vi "PosStrikerAnguloGolV1.vi"(8 "AnguloAttacker":dbl, 9 "atacando contra":bool, 10 "IA State":T1={"our_robots"=[], "enemy_robots"=[], "balls"=[], "geometry"={"line_width"=0, "field_length"=0, "field_width"=0, "boundary_width"=0, "referee_width"=0, "goal_width"=0, "goal_depth"=0, "goal_wall_width"=0, "center_circle_radius"=0, "defense_radius"=0, "defense_stretch"=0, "free_kick_from_defense_dist"=0, "penalty_spot_from_field_line_dist"=0, "penalty_line_from_spot_dist"=0}, "IA Judge"={"stage"="", "command"="", "our_goalie_id"=0.0, "enemy_goalie_id"=0.0, "command enum"=enum."Halt", "Time"=enum."Azul"}, "Received Timestamp"=timestamp(0 s since 1904-01-01), "Events"={"Touch"=FALSE, "Ball out"=FALSE, "id touch"=0.0, "Ball out of \nVision"=FALSE, "Ball inside \nGoalie area"=FALSE, "Robot not responding"=FALSE, "Robots responding status"=[1.0, 1.0, 1.0, 1.0, 1.0, 1.0], "Enemy Ball \nPossession"=FALSE, "Pass State"=FALSE, "id end of pass"=0.0, "Kick"=FALSE, "Id ini Possession"=0.0, "Ball Possesion"=FALSE, "Id Possesion"=0.0, "Direct Kick"=FALSE, "2nd Strk Ativo"=FALSE}}) -> (2 "theta final":dbl)   [LabVIEW 2017]
uses:
  Core/AI Input.ctl
  Core/AI Robot.ctl
  Intel/Functions Enum.ctl
  Intel/AttackerStates.ctl
  Path Planning/RRT/PathDests.ctl
  Path Planning/RRT/PathDest.ctl
  Core/AI Ball.ctl
  Core/Field Size.ctl
  Core/AI Judge.ctl
  Intel/Command Enum.ctl
  Events/Events.ctl
panel:
  in  "XdoAttacker":dbl
  in  "YdoAttacker":dbl
  in  "Array":dbl[](array[numeric])=[0.0, 0.0, 0.0, 0.0, 0.0, 0.0]
  in  "Contador 2":dbl
  in  "theta2":dbl=-1.57
  in  "inicio do intervalo":dbl=-1.57
  in  "tamanho do intervalo":dbl
  in  "valor de theta":dbl
  in  "RobôsParaAnalisar":dbl[][](array[numeric])=[[99999.0, 99999.0], [99999.0, 99999.0], [99999.0, 99999.0], [99999.0, 99999.0], [99999.0, 99999.0], [99999.0, 99999.0], [99999.0, 99999.0]]
  in  "Contador":dbl
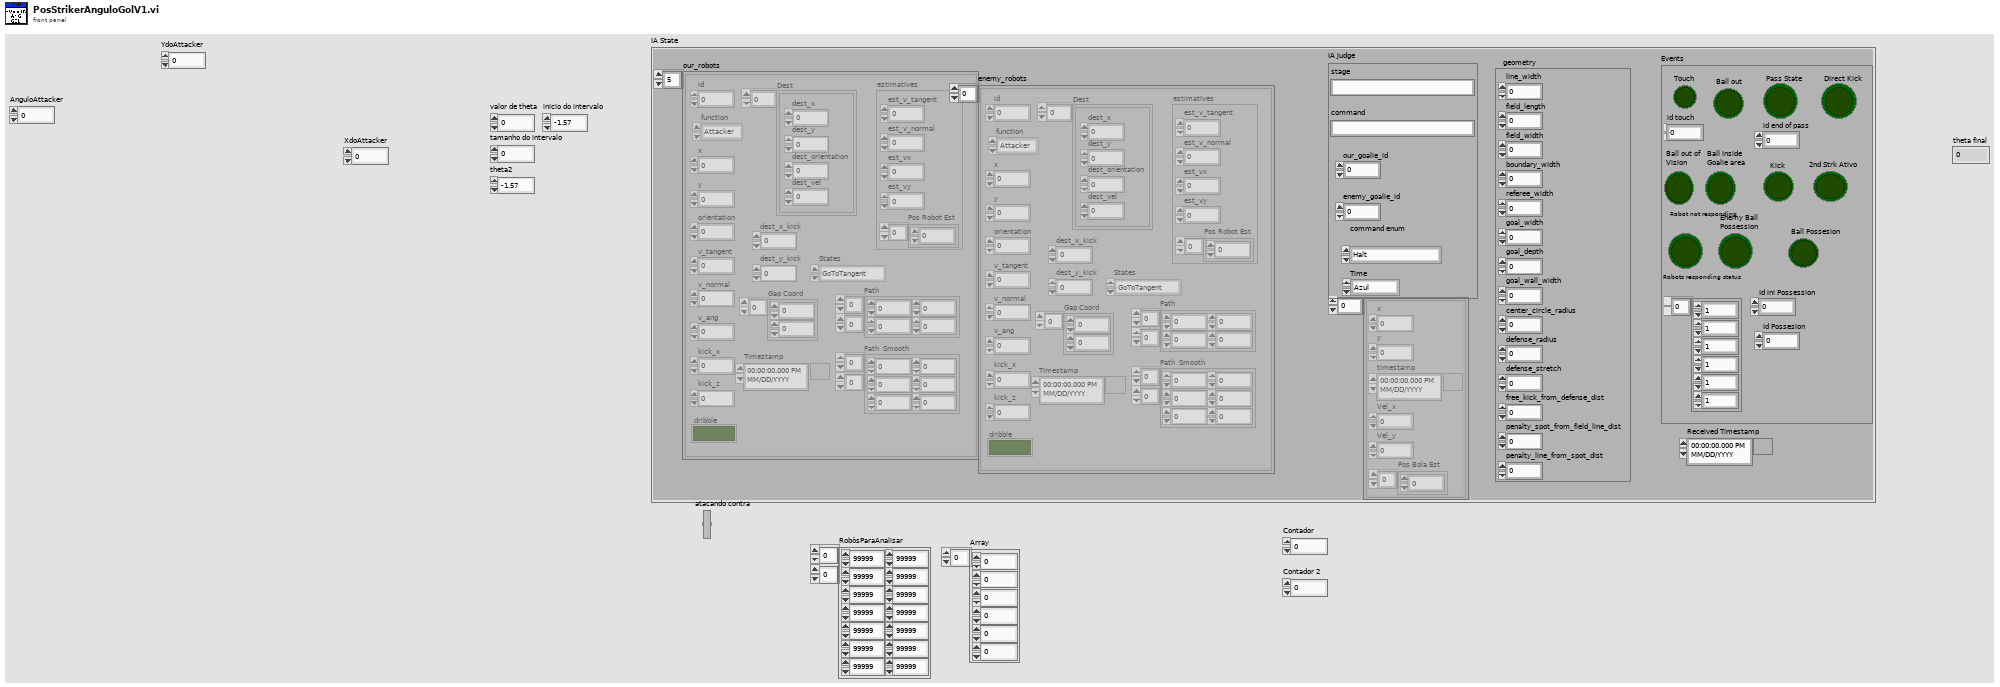
[diagram p1: front panel]
types:
  T1 = typedef "AI Input.ctl" = cluster{"our_robots":T2[], "enemy_robots":T2[], "balls":T7[], "geometry":T8, "IA Judge":T9, "Received Timestamp":timestamp, "Events":T11}
  T2 = typedef "AI Robot.ctl" = cluster{"id":u32, "function":T3, "x":dbl, "y":dbl, "orientation":dbl, "v_tangent":dbl, "v_normal":dbl, "v_ang":dbl, "kick_x":dbl, "kick_z":dbl, "dribble":bool, "Timestamp":timestamp, "estimatives":cluster{"est_v_tangent":dbl, "est_v_normal":dbl, "est_vx":dbl, "est_vy":dbl, "Pos Robot Est":dbl[]}, "dest_x_kick":dbl, "dest_y_kick":dbl, "Gap Coord":dbl[], "States":T4, "Path ":dbl[][], "Path  Smooth":dbl[][], "Dest":T5}
  T3 = typedef "Functions Enum.ctl" = enum16{"2nd Striker", "Attacker", "Goalie", "Defender", "Striker", "Goto 0", "Dummy", "Kicker", "ZigZag 0", "ZigZag 1", "ZigZag 2", "ZigZag 3", "ZigZag 4", "ZigZag 5", "ZigZag 6", "ZigZag 7", "ZigZag 8", ""}
  T4 = typedef "AttackerStates.ctl" = enum16{"Pass", "GoToTangent", "BallGetting", "GoToKick", ""}
  T5 = typedef "PathDests.ctl" = T6[]
  T6 = typedef "PathDest.ctl" = cluster{"dest_x":dbl, "dest_y":dbl, "dest_orientation":dbl, "dest_vel":dbl}
  T7 = typedef "AI Ball.ctl" = cluster{"x":dbl, "y":dbl, "timestamp":timestamp, "Vel_x":dbl, "Vel_y":dbl, "Pos Bola Est":dbl[]}
  T8 = typedef "Field Size.ctl" = cluster{"line_width":u32, "field_length":u32, "field_width":u32, "boundary_width":u32, "referee_width":u32, "goal_width":u32, "goal_depth":u32, "goal_wall_width":u32, "center_circle_radius":u32, "defense_radius":u32, "defense_stretch":u32, "free_kick_from_defense_dist":u32, "penalty_spot_from_field_line_dist":u32, "penalty_line_from_spot_dist":u32}
  T9 = typedef "AI Judge.ctl" = cluster{"stage":string, "command":string, "our_goalie_id":dbl, "enemy_goalie_id":dbl, "command enum":T10, "Time":enum16{"Azul", "Amarelo"}}
  T10 = typedef "Command Enum.ctl" = enum16{"Halt", "Stop", "Force Start", "PKA Normal Start", "Prepare Kickoff Ally", "PKE Normal Start", "Prepare Kickoff Enemy", "Prepare Penalty Ally", "PPA Normal Start", "Prepare Penalty Enemy", "PPE Normal Start", "Direct Free Enemy", "Direct Free Ally", "Indirect Free Enemy", "Indirect Free Ally", "Timeout Enemy", "Timeout Ally", "Goal Enemy", "Goal Ally", "Ball Placement Enemy", "Ball Placement Ally", "Normal Half Time", "Extra Time Break", "Extra Half Time", "None", "Post Game"}
  T11 = typedef "Events.ctl" = cluster{"Touch":bool, "Ball out":bool, "id touch":dbl, "Ball out of \nVision":bool, "Ball inside \nGoalie area":bool, "Robot not responding":bool, "Robots responding status":dbl[], "Enemy Ball \nPossession":bool, "Pass State":bool, "id end of pass":dbl, "Kick":bool, "Id ini Possession":dbl, "Ball Possesion":bool, "Id Possesion":dbl, "Direct Kick":bool, "2nd Strk Ativo":bool}
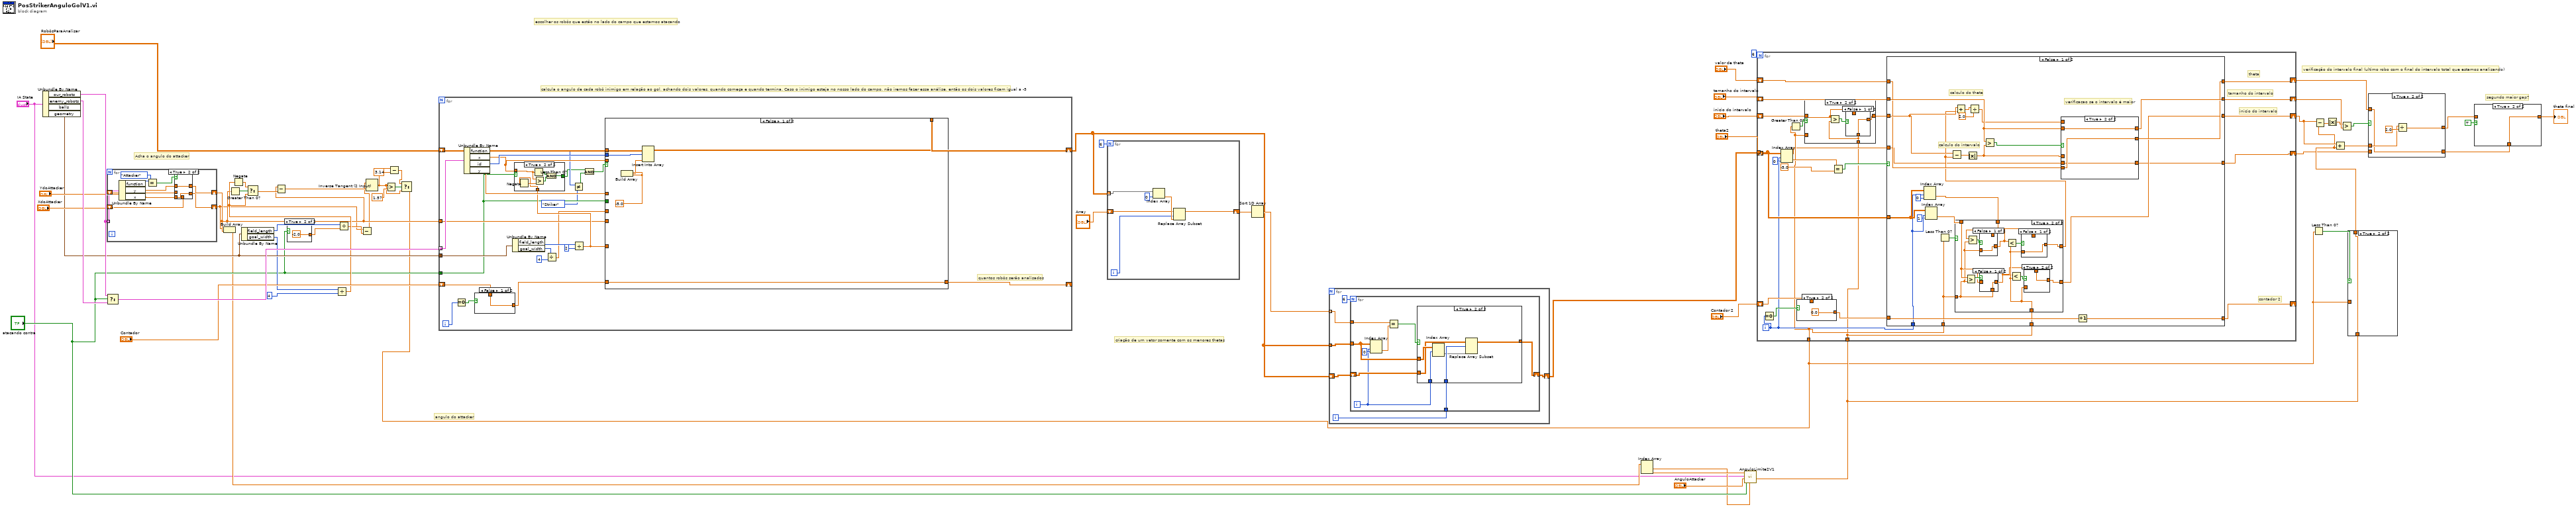
[diagram p0: block diagram]
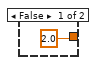
[diagram p4: hidden frame]
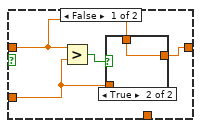
[diagram p8: hidden frame]
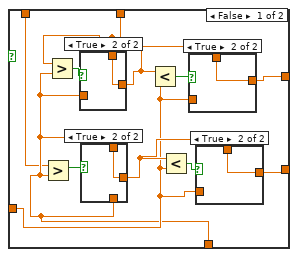
[diagram p12: hidden frame]
diagram:
  # "segundo maior gap?"
  # "verificação do intervalo final (ultimo robo com o final do intervalo total que estamos analisando)"
  # "calcula o angulo de cada robô inimigo em relação ao gol, achando dois valores, quando começa e quando termina. Caso o inimigo esteja no nosso lado do campo, não iremos fazer essa análise, então os dois valores ficam igual a -5"
  # "angulo do attacker"
  # "Acha o angulo do attacker"
  # "criação de um vetor somente com os menores thetas"
  # "escolher os robôs que estão no lado do campo que estamos atacando"
  n1 = Unbundle By Name("IA State") -> ("our_robots"=w37:T2[], "enemy_robots"=w60:T2[], "geometry"=w34:T8)  [unwired: 1 out]
  n2 = for {
    tunnel: w37 -> [w70] mode=indexing
    shift-right: [w65] -> w15
    shift-left: "YdoAttacker" -> [w64]
    shift-right: [w62] -> w14
    shift-left: "XdoAttacker" -> [w61]
    n3 = Unbundle By Name(w70) -> ("function"=w69:T3, "y"=w66:dbl, "x"=w63:dbl)
    n4 = Equal?(x=w69, y=Functions_Enum."Attacker") -> (x = y?=w67:bool)
    n5 = case shown="True" w67 {
      tunnel: w66 -> [_ w74]
      tunnel: [w72 w74] -> w65
      tunnel: w64 -> [w72 _]
      tunnel: w63 -> [_ w73]
      tunnel: [w71 w73] -> w62
      tunnel: w61 -> [w71 _]
      frame False {
      }
      frame True {
      }
    }
  }
  n6 = Select(t=w37, s="atacando contra", f=w60) -> (s? t:f=w59:T2[])
  n7 = Build Array(w14, w15) -> (w13:dbl[])
  n8 = Greater Than 0?(x=w15) -> (x > 0?=w30:bool)
  n9 = Unbundle By Name(w34) -> ("field_length"=w31:u32, "goal_width"=w33:u32)
  n10 = case shown="True" "atacando contra" {
    tunnel: [2.0 ("y") -2.0 ("y")] -> w25
    frame False {
    }
    frame True {
    }
  }
  n11 = Divide(x=w33, y=u32 4) -> (x/y=w28:dbl)
  n12 = Negate(x=w28) -> (-x=w29:dbl)
  n13 = Select(t=w29, s=w30, f=w28) -> (s? t:f=w27:dbl)
  n14 = Subtract(x=w15, y=w27) -> (x-y=w2:dbl)
  n15 = Divide(x=w31, y=w25) -> (x/y=w26:dbl)
  n16 = Subtract(x=w14, y=w26) -> (x-y=w1:dbl)
  n17 = Inverse Tangent (2 Input)(1:w2, 2:w1) -> (0:w4:dbl)
  n18 = Greater?(x=w4, y=1.57) -> (0:w7:bool)
  n19 = Subtract(x=w4, y=3.14) -> (x-y=w5:dbl)
  n20 = Select(t=w5, s=w7, f=w4) -> (s? t:f=w3:dbl)
  n21 = for {
    tunnel: w59 -> [w101] mode=indexing
    tunnel: "atacando contra" -> [w83]
    shift-right: [w91] -> w47
    shift-left: "RobôsParaAnalisar" -> [w100]
    shift-right: [w92] -> _
    shift-left: "Contador" -> [w94]
    tunnel: w34 -> [w84]
    tunnel: w15 -> [w88]
    i -> [w95]
    # "quantos robôs serão analisados"
    n22 = Equal To 0?(x=w95) -> (x = 0?=w96:bool)
    n23 = Unbundle By Name(w101) -> ("function"=w81:T3, "x"=w98:dbl, "id"=w99:u32, "y"=w97:dbl)
    n24 = case shown="False" w96 {
      tunnel: w94 -> [w102 _]
      tunnel: [w102 0.0] -> w93
      frame False {
      }
      frame True {
      }
    }
    n25 = Unbundle By Name(w84) -> ("field_length"=w90:u32, "goal_width"=w87:u32)
    n26 = Divide(x=w87, y=u32 4) -> (x/y=w85:dbl)
    n27 = Not Equal?(x=w81, y=Functions_Enum."Striker") -> (x != y?=w78:bool)
    n28 = Divide(x=w90, y=u32 2) -> (x/y=w89:dbl)
    n29 = case shown="True" w83 {
      tunnel: w98 -> [w108 w109]
      tunnel: [w104 w114] -> w77
      tunnel: w89 -> [w107 w110]
      frame False {
        n30 = Less?(x=w108, y=w107) -> (x < y?=w105:bool)
        n31 = Greater Than 0?(x=w108) -> (x > 0?=w106:bool)
        n32 = And(x=w106, y=w105) -> (x .and. y?=w104:bool)
      }
      frame True {
        n33 = Negate(x=w110) -> (-x=w111:dbl)
        n34 = Less Than 0?(x=w109) -> (x < 0?=w113:bool)
        n35 = Greater?(x=w109, y=w111) -> (0:w112:bool)
        n36 = And(x=w113, y=w112) -> (x .and. y?=w114:bool)
      }
    }
    n37 = And(x=w77, y=w78) -> (x .and. y?=w79:bool)
    n38 = case shown="False" w79 {
      tunnel: w100 -> [w119 w126]
      tunnel: w99 -> [w118 w124]
      tunnel: w98 -> [_ w128]
      tunnel: w97 -> [_ w125]
      tunnel: w93 -> [w120 w130]
      tunnel: [w120 w131] -> w92
      tunnel: [w115 w123] -> w91
      tunnel: w83 -> [_ w129]
      tunnel: w89 -> [_ w127]
      tunnel: w88 -> [_ w122]
      tunnel: w85 -> [_ w121]
      frame False {
        w117 = -5.0 ("element")
        n39 = Build Array(w117, w117) -> (w116:dbl[])
        n40 = Insert Into Array(array=w119, index (row)=w118, new element=w116) -> (w115:dbl[][])  [unwired: 1 in]
      }
      frame True {
        n41 = case shown="False" w129 {
          tunnel: w128 -> [w143 w191]
          tunnel: w127 -> [w142 w194]
          tunnel: w126 -> [w144 w186]
          tunnel: w125 -> [w135 w175]
          tunnel: w124 -> [w145 w185]
          tunnel: [w141 w182] -> w123
          tunnel: w122 -> [w134 w179]
          tunnel: w121 -> [w133 w176]
          frame False {
            # "y"
            # "x"
            n42 = Add(x=w143, y=90.0) -> (x+y=w151:dbl)
            n43 = Less Than 0?(x=w134) -> (x < 0?=w138:bool)
            n44 = Negate(x=w133) -> (-x=w137:dbl)
            n45 = Select(t=w133, s=w138, f=w137) -> (s? t:f=w136:dbl)
            n46 = Subtract(x=w135, y=w136) -> (x-y=w132:dbl)
            n47 = Greater?(x=w151, y=w142) -> (0:w152:bool)
            n48 = Subtract(x=w143, y=90.0) -> (x-y=w149:dbl)
            n49 = case shown="False" w152 {
              tunnel: w151 -> [w171 _]
              tunnel: [w168 1.57] -> w147
              tunnel: w142 -> [w170 _]
              tunnel: w132 -> [w169 _]
              frame False {
                n50 = Subtract(x=w171, y=w170) -> (x-y=w167:dbl)
                n51 = Absolute Value(x=w167) -> (abs(x)=w166:dbl)
                n52 = Inverse Tangent (2 Input)(1:w166, 2:w169) -> (0:w168:dbl)
              }
              frame True {
              }
            }
            n53 = Subtract(x=w149, y=w142) -> (x-y=w139:dbl)
            n54 = Absolute Value(x=w139) -> (abs(x)=w140:dbl)
            n55 = Inverse Tangent (2 Input)(1:w140, 2:w135) -> (0:w146:dbl)
            n56 = Greater?(x=w147, y=w146) -> (0:w148:bool)
            n57 = case shown="True" w148 {
              tunnel: w144 -> [w156 w162]
              tunnel: w145 -> [w158 w165]
              tunnel: w147 -> [w155 w163]
              tunnel: w146 -> [w157 w161]
              tunnel: [w154 w160] -> w141
              frame False {
                n58 = Build Array(w157, w155) -> (w159:dbl[])
                n59 = Insert Into Array(array=w156, index (row)=w158, new element=w159) -> (w154:dbl[][])  [unwired: 1 in]
              }
              frame True {
                n60 = Build Array(w163, w161) -> (w164:dbl[])
                n61 = Insert Into Array(array=w162, index (row)=w165, new element=w164) -> (w160:dbl[][])  [unwired: 1 in]
              }
            }
          }
          frame True {
            # "y"
            # "x"
            n62 = Negate(x=w194) -> (-x=w188:dbl)
            n63 = Subtract(x=w191, y=90.0) -> (x-y=w192:dbl)
            n64 = Greater Than 0?(x=w179) -> (x > 0?=w178:bool)
            n65 = Negate(x=w176) -> (-x=w177:dbl)
            n66 = Select(t=w176, s=w178, f=w177) -> (s? t:f=w174:dbl)
            n67 = Subtract(x=w175, y=w174) -> (x-y=w173:dbl)
            n68 = Less?(x=w192, y=w188) -> (x < y?=w193:bool)
            n69 = Add(x=w191, y=90.0) -> (x+y=w189:dbl)
            n70 = case shown="False" w193 {
              tunnel: w192 -> [w213 _]
              tunnel: [w210 1.57] -> w184
              tunnel: w188 -> [w212 _]
              tunnel: w173 -> [w211 _]
              frame False {
                n71 = Subtract(x=w213, y=w212) -> (x-y=w208:dbl)
                n72 = Absolute Value(x=w208) -> (abs(x)=w209:dbl)
                n73 = Inverse Tangent (2 Input)(1:w209, 2:w211) -> (0:w210:dbl)
              }
              frame True {
              }
            }
            n74 = Subtract(x=w189, y=w188) -> (x-y=w180:dbl)
            n75 = Absolute Value(x=w180) -> (abs(x)=w181:dbl)
            n76 = Inverse Tangent (2 Input)(1:w181, 2:w175) -> (0:w183:dbl)
            n77 = Greater?(x=w184, y=w183) -> (0:w187:bool)
            n78 = case shown="True" w187 {
              tunnel: w186 -> [w198 w204]
              tunnel: w185 -> [w200 w207]
              tunnel: w184 -> [w197 w205]
              tunnel: w183 -> [w199 w203]
              tunnel: [w196 w202] -> w182
              frame False {
                n79 = Build Array(w199, w197) -> (w201:dbl[])
                n80 = Insert Into Array(array=w198, index (row)=w200, new element=w201) -> (w196:dbl[][])  [unwired: 1 in]
              }
              frame True {
                n81 = Build Array(w205, w203) -> (w206:dbl[])
                n82 = Insert Into Array(array=w204, index (row)=w207, new element=w206) -> (w202:dbl[][])  [unwired: 1 in]
              }
            }
          }
        }
        n83 = Increment(x=w130) -> (x+1=w131:dbl)
      }
    }
  }
  n84 = for {
    N: 6 -> [_]
    tunnel: w47 -> [w220] mode=indexing
    shift-right: [w215] -> w49
    shift-left: "Array" -> [w216]
    i -> [w217]
    n85 = Index Array(array=w220, index=0) -> (element=w218:dbl)
    n86 = Replace Array Subset(array=w216, new element=w218, index=w217) -> (w215:dbl[])
  }
  n87 = Sort 1D Array(array=w49) -> (sorted array=w48:dbl[])
  n88 = for {
    tunnel: w48 -> [w223] mode=indexing
    tunnel: w47 -> [w225]
    shift-right: [w221] -> w46
    shift-left: w47 -> [w224]
    i -> [w222]
    n89 = for {
      N: 6 -> [_]
      tunnel: w225 -> [w231]
      shift-right: [w227] -> w221
      shift-left: w224 -> [w230]
      tunnel: w223 -> [w233]
      tunnel: w222 -> [w228]
      i -> [w229]
      n90 = Index Array(array=w231, index (row)=w229, index (col)=0 ("disabled index (col)")) -> (element=w234:dbl)
      n91 = Equal?(x=w233, y=w234) -> (x = y?=w232:bool)
      n92 = case shown="True" w232 {
        tunnel: w231 -> [_ w242]
        tunnel: w230 -> [w236 w238]
        tunnel: w229 -> [_ w241]
        tunnel: w228 -> [_ w240]
        tunnel: [w236 w237] -> w227
        frame False {
        }
        frame True {
          n93 = Index Array(array=w242, index (row)=w241) -> (element=w239:dbl[])  [unwired: 1 in]
          n94 = Replace Array Subset(array=w238, new element=w239, index (row)=w240) -> (w237:dbl[][])  [unwired: 1 in]
        }
      }
    }
  }
  n95 = Index Array(array=w13) -> (element #1=w11:dbl, element #2=w12:dbl)  [unwired: 2 in]
  n96 = call "AnguloLimite2V1.vi"("XdoAttacker"=w11, "atacando contra"="atacando contra", "AnguloAttacker"="AnguloAttacker", "IA State"="IA State", "YdoAttacker"=w12) -> ("Angulo Limite"=w9:dbl)  [unwired: 6 in]
  n97 = for {
    N: 6 -> [_]
    tunnel: w46 -> [w253]
    shift-right: [w261] -> w43
    shift-left: "valor de theta" -> [w262]
    shift-right: [w259] -> w45
    shift-left: "tamanho do intervalo" -> [w260]
    shift-right: [w258] -> w40
    shift-left: "inicio do intervalo" -> [w247]
    shift-right: [w254] -> _
    shift-left: "Contador 2" -> [w256]
    tunnel: w3 -> [w246]
    shift-right: [w244] -> w22
    shift-left: "theta2" -> [w245]
    tunnel: w9 -> [w243]
    i -> [w252]
    # "contador 2"
    # "inicio do intervalo"
    # "tamanho do intervalo"
    # "theta"
    n98 = Equal To 0?(x=w252) -> (x = 0?=w257:bool)
    n99 = Index Array(array=w253, index (row)=w252, index (col)=0 ("disabled index (col)")) -> (element=w251:dbl)
    n100 = Greater Than 0?(x=w246) -> (x > 0?=w249:bool)
    n101 = case shown="True" w257 {
      tunnel: w256 -> [w277 _]
      tunnel: [w277 0.0] -> w255
      frame False {
      }
      frame True {
      }
    }
    n102 = case shown="True" w249 {
      tunnel: [w267 w271] -> w248
      tunnel: w247 -> [w266 w273]
      tunnel: w246 -> [w265 _]
      tunnel: w243 -> [_ w272]
      frame False {
        n103 = Greater?(x=w266, y=w265) -> (0:w268:bool)
        n104 = case shown="True" w268 {
          tunnel: [w269 w270] -> w267
          tunnel: w266 -> [_ w270]
          tunnel: w265 -> [w269 _]
          frame False {
          }
          frame True {
          }
        }
      }
      frame True {
        n105 = Greater?(x=w273, y=w272) -> (0:w274:bool)
        n106 = case shown="False" w274 {
          tunnel: [w275 w276] -> w271
          tunnel: w273 -> [_ w276]
          tunnel: w272 -> [w275 _]
          frame False {
          }
          frame True {
          }
        }
      }
    }
    n107 = Equal?(x=w251, y=-5.0) -> (x = y?=w250:bool)
    n108 = case shown="False" w250 {
      tunnel: w262 -> [w288 w355]
      tunnel: [w289 w355] -> w261
      tunnel: w260 -> [w293 w354]
      tunnel: [w292 w354] -> w259
      tunnel: w248 -> [w304 w353]
      tunnel: [w282 w353] -> w258
      tunnel: w255 -> [w302 w352]
      tunnel: [w303 w352] -> w254
      tunnel: w253 -> [w301 _]
      tunnel: w252 -> [w300 _]
      tunnel: w246 -> [w286 _]
      tunnel: w245 -> [w281 w351]
      tunnel: [w280 w351] -> w244
      tunnel: w243 -> [w279 _]
      frame False {
        # "calculo do theta"
        # "calculo do intervalo"
        # "verificacao se o intervalo é maior"
        n109 = Index Array(array=w301, index (row)=w300, index (col)=0 ("disabled index (col)")) -> (element=w285:dbl)
        n110 = Index Array(array=w301, index (row)=w300, index (col)=1 ("disabled index (col)")) -> (element=w283:dbl)
        n111 = Less Than 0?(x=w286) -> (x < 0?=w287:bool)
        n112 = case shown="True" w287 {
          tunnel: w283 -> [w305 w333]
          tunnel: w285 -> [w306 w335]
          tunnel: w286 -> [w311 w332]
          tunnel: [w310 w330] -> w284
          tunnel: [w309 w326] -> w282
          tunnel: w279 -> [w308 w327]
          frame False {
            n113 = Greater?(x=w305, y=w308) -> (0:w315:bool)
            n114 = Greater?(x=w306, y=w308) -> (0:w316:bool)
            n115 = case shown="True" w316 {
              tunnel: [w323 w324] -> w307
              tunnel: w308 -> [w323 _]
              tunnel: w306 -> [_ w324]
              frame False {
              }
              frame True {
              }
            }
            n116 = case shown="True" w315 {
              tunnel: [w321 w322] -> w312
              tunnel: w308 -> [w321 _]
              tunnel: w308 -> [_ w322]
              frame False {
              }
              frame True {
              }
            }
            n117 = Less?(x=w307, y=w311) -> (x < y?=w314:bool)
            n118 = Less?(x=w312, y=w311) -> (x < y?=w313:bool)
            n119 = case shown="True" w314 {
              tunnel: [w319 w320] -> w310
              tunnel: w311 -> [w319 _]
              tunnel: w307 -> [_ w320]
              frame False {
              }
              frame True {
              }
            }
            n120 = case shown="True" w313 {
              tunnel: [w317 w318] -> w309
              tunnel: w312 -> [_ w318]
              tunnel: w311 -> [w317 _]
              frame False {
              }
              frame True {
              }
            }
          }
          frame True {
            n121 = Greater?(x=w333, y=w332) -> (0:w334:bool)
            n122 = Greater?(x=w335, y=w332) -> (0:w336:bool)
            n123 = case shown="False" w336 {
              tunnel: [w343 w344] -> w329
              tunnel: w335 -> [_ w344]
              tunnel: w332 -> [w343 _]
              frame False {
              }
              frame True {
              }
            }
            n124 = case shown="False" w334 {
              tunnel: w333 -> [_ w342]
              tunnel: [w341 w342] -> w325
              tunnel: w332 -> [w341 _]
              frame False {
              }
              frame True {
              }
            }
            n125 = Less?(x=w329, y=w327) -> (x < y?=w331:bool)
            n126 = Less?(x=w325, y=w327) -> (x < y?=w328:bool)
            n127 = case shown="False" w331 {
              tunnel: [w339 w340] -> w330
              tunnel: w329 -> [_ w340]
              tunnel: w327 -> [w339 _]
              frame False {
              }
              frame True {
              }
            }
            n128 = case shown="True" w328 {
              tunnel: [w337 w338] -> w326
              tunnel: w325 -> [_ w338]
              tunnel: w327 -> [w337 _]
              frame False {
              }
              frame True {
              }
            }
          }
        }
        n129 = Subtract(x=w304, y=w284) -> (x-y=w297:dbl)
        n130 = Add(x=w304, y=w284) -> (x+y=w296:dbl)
        n131 = Absolute Value(x=w297) -> (abs(x)=w291:dbl)
        n132 = Divide(x=w296, y=2.0) -> (x/y=w290:dbl)
        n133 = Greater?(x=w293, y=w291) -> (0:w294:bool)
        n134 = case shown="True" w294 {
          tunnel: w293 -> [_ w350]
          tunnel: [w347 w350] -> w292
          tunnel: w291 -> [w347 _]
          tunnel: w288 -> [w345 w349]
          tunnel: w290 -> [w346 _]
          tunnel: [w346 w349] -> w289
          tunnel: w281 -> [_ w348]
          tunnel: [w345 w348] -> w280
          frame False {
          }
          frame True {
          }
        }
        n135 = Increment(x=w302) -> (x+1=w303:dbl)
      }
      frame True {
      }
    }
  }
  n136 = Less Than 0?(x=w3) -> (x < 0?=w24:bool)
  n137 = case shown="True" w24 {
    tunnel: [w356 w357] -> w39
    tunnel: w3 -> [w356 _]
    tunnel: w9 -> [_ w357]
    frame False {
    }
    frame True {
    }
  }
  n138 = Subtract(x=w40, y=w39) -> (x-y=w42:dbl)
  n139 = Absolute Value(x=w42) -> (abs(x)=w41:dbl)
  n140 = Add(x=w40, y=w39) -> (x+y=w38:dbl)
  n141 = Greater?(x=w41, y=w45) -> (0:w44:bool)
  n142 = case shown="True" w44 {
    tunnel: [w359 w362] -> w18
    tunnel: w43 -> [w359 w360]
    tunnel: w38 -> [_ w361]
    tunnel: w22 -> [w358 _]
    tunnel: [w358 w360] -> w19
    frame False {
    }
    frame True {
      n143 = Divide(x=w361, y=2.0) -> (x/y=w362:dbl)
    }
  }
  n144 = case shown="True" TRUE {
    tunnel: [w364 w365] -> w20
    tunnel: w19 -> [_ w365]
    tunnel: w18 -> [w364 _]
    frame False {
    }
    frame True {
    }
  }
  "theta final" <- w20
